vi "vaj timing control(new).vi"(8 "Error In":errorcluster, 10 "VAJ":cluster{"V":dbl, "A":dbl, "J":dbl}, 11 "D":dbl) -> (0 "Error Out":errorcluster, 3 "Array":cluster{"Numeric":dbl, "Numeric":dbl}[](array[cluster]))   [LabVIEW 2019]
uses:
  fd133df4-cac8-46f0-a5d4-c7e4d07d299a.vi
  2734163e-cfed-4914-b593-cf69aa2ffa15.vi
  <vilib>/Utility/error.llb/Error Cluster From Error Code.vi
  <vilib>/ErrorRing/Error Ring.xnode
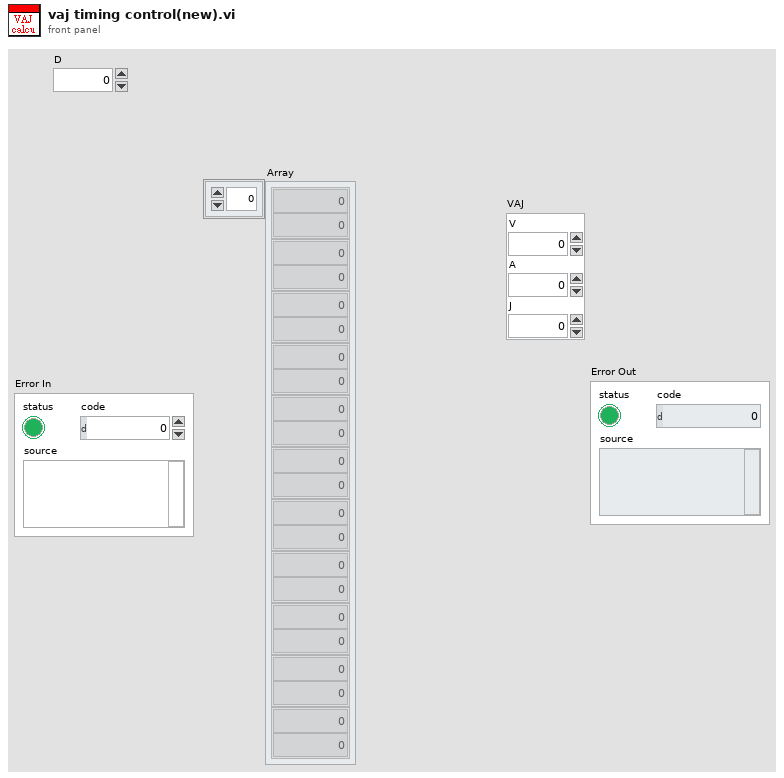
[diagram p1: front panel]
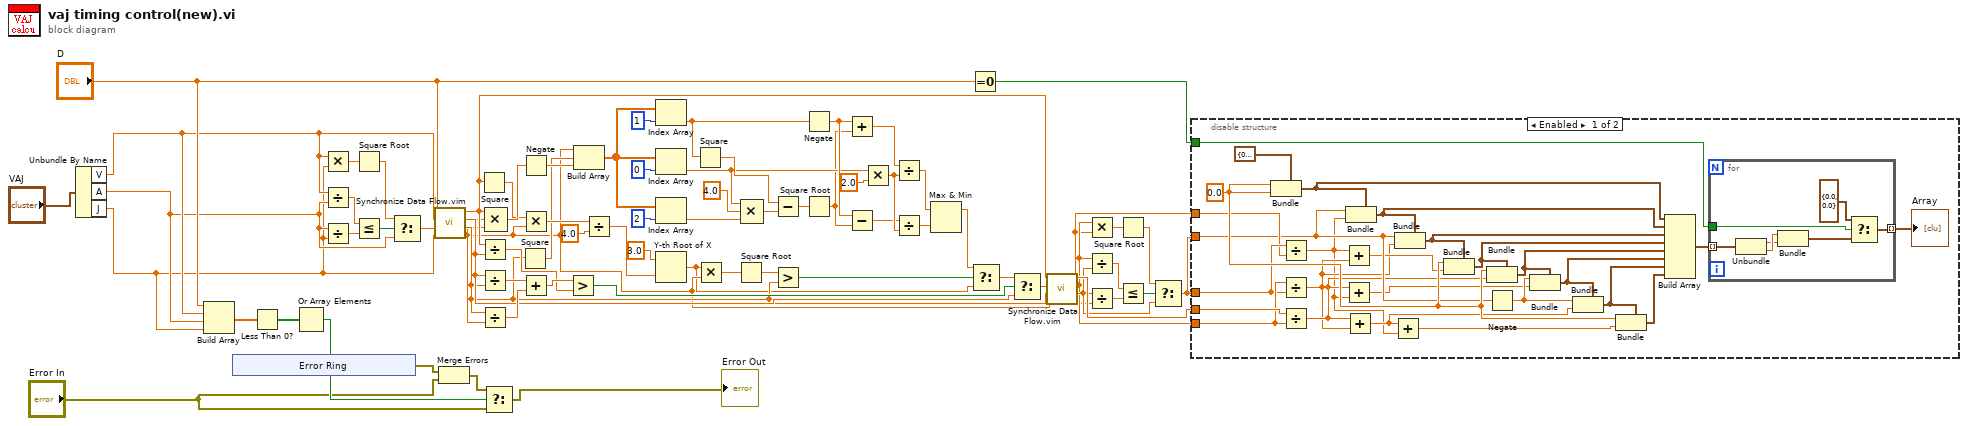
[diagram p0: block diagram]
diagram:
  n1 = Unbundle By Name("VAJ") -> ("V"=w10:dbl, "A"=w9:dbl, "J"=w8:dbl)
  n2 = Build Array("D", w10, w9, w8) -> (w7:dbl[])
  n3 = xnode "Error Ring"() -> ("error out"=w4:errorcluster)
  n4 = Less Than 0?(x=w7) -> (x < 0?=w6:bool[])
  n5 = Or Array Elements(Boolean array=w6) -> (logical OR=w5:bool)
  n6 = Multiply(x=w10, y=w8) -> (x*y=w69:dbl)
  n7 = Divide(x=w10, y=w9) -> (x/y=w72:dbl)
  n8 = Divide(x=w9, y=w8) -> (x/y=w71:dbl)
  n9 = Square Root(x=w69) -> (sqrt(x)=w68:dbl)
  n10 = Less Or Equal?(x=w72, y=w71) -> (x <= y?=w70:bool)
  n11 = Select(t=w68, s=w70, f=w9) -> (s? t:f=w67:dbl)
  n12 = call "Synchronize Data Flow.vim"("input 4"=w8, "input 3"=w67, "input 2"=w10, "input 1"="D") -> ("output 4"=w17:dbl, "output 3"=w18:dbl, "output 2"=w61:dbl, "output 1"=w29:dbl)
  n13 = Merge Errors(w4, "Error In") -> (w3:errorcluster)
  n14 = Square(x=w29) -> (x^2=w28:dbl)
  n15 = Divide(x=w29, y=w61) -> (x/y=w63:dbl)
  n16 = Divide(x=w61, y=w18) -> (x/y=w65:dbl)
  n17 = Divide(x=w18, y=w17) -> (x/y=w66:dbl)
  n18 = Select(t=w3, s=w5, f="Error In") -> (s? t:f=→"Error Out":errorcluster)
  n19 = Compound Arithmetic op=MULTIPLY(w29, w18, w17) -> (w60:dbl)
  n20 = Square(x=w18) -> (x^2=w19:dbl)
  n21 = Negate(x=w60) -> (-x=w59:dbl)
  n22 = Multiply(x=w28, y=w17) -> (x*y=w27:dbl)
  n23 = Add(x=w65, y=w66) -> (x+y=w64:dbl)
  n24 = Greater?(x=w64, y=w63) -> (0:w62:bool)
  n25 = Build Array(w17, w19, w59) -> (w55:dbl[])
  n26 = Divide(x=w27, y=4.0) -> (x/y=w25:dbl)
  n27 = Index Array(array=w55, index=1) -> (element=w49:dbl)
  n28 = Index Array(array=w55, index=0) -> (element=w46:dbl)
  n29 = Index Array(array=w55, index=2) -> (element=w45:dbl)
  n30 = Y-th Root of X(1:w25, 2:3.0 ("y")) -> (0:w16:dbl)
  n31 = Square(x=w49) -> (x^2=w48:dbl)
  n32 = Multiply(x=w16, y=w17) -> (x*y=w23:dbl)
  n33 = Square Root(x=w23) -> (sqrt(x)=w22:dbl)
  n34 = Compound Arithmetic op=MULTIPLY(w46, 4.0 ("value"), w45) -> (w47:dbl)
  n35 = Subtract(x=w48, y=w47) -> (x-y=w43:dbl)
  n36 = Greater?(x=w22, y=w18) -> (0:w21:bool)
  n37 = Negate(x=w49) -> (-x=w52:dbl)
  n38 = Square Root(x=w43) -> (sqrt(x)=w39:dbl)
  n39 = Add(x=w52, y=w39) -> (x+y=w51:dbl)
  n40 = Subtract(x=w52, y=w39) -> (x-y=w50:dbl)
  n41 = Multiply(x=w46, y=2.0) -> (x*y=w53:dbl)
  n42 = Divide(x=w51, y=w53) -> (x/y=w42:dbl)
  n43 = Divide(x=w50, y=w53) -> (x/y=w41:dbl)
  n44 = Max & Min(x=w42, y=w41) -> (max(x,y)=w20:dbl)  [unwired: 1 out]
  n45 = Equal To 0?(x="D") -> (x = 0?=w13:bool)
  n46 = Select(t=w20, s=w21, f=w16) -> (s? t:f=w15:dbl)
  n47 = Select(t=w15, s=w62, f=w61) -> (s? t:f=w14:dbl)
  n48 = call "Synchronize Data Flow.vim"("input 4"=w17, "input 3"=w18, "input 2"=w14, "input 1"=w29) -> ("output 4"=w31:dbl, "output 3"=w33:dbl, "output 2"=w32:dbl, "output 1"=w40:dbl)
  n49 = Multiply(x=w32, y=w31) -> (x*y=w35:dbl)
  n50 = Divide(x=w32, y=w33) -> (x/y=w38:dbl)
  n51 = Divide(x=w33, y=w31) -> (x/y=w37:dbl)
  n52 = Square Root(x=w35) -> (sqrt(x)=w34:dbl)
  n53 = Less Or Equal?(x=w38, y=w37) -> (x <= y?=w36:bool)
  n54 = Select(t=w34, s=w36, f=w33) -> (s? t:f=w30:dbl)
  n55 = disable-structure shown="Enabled" {
    disable-tunnel: w40 -> [w86 _]
    disable-tunnel: w32 -> [w85 _]
    disable-tunnel: w30 -> [w84 _]
    disable-tunnel: w31 -> [w83 _]
    disable-tunnel: w30 -> [w82 _]
    disable-tunnel: w13 -> [w73 _]
    frame Enabled {
      w95 = 0.0
      n56 = Bundle(cluster=cluster{dbl, dbl} {0.0, 0.0} ("output cluster"), w95, w95) -> (w93:cluster{dbl, dbl})
      n57 = Divide(x=w84, y=w83) -> (x/y=w74:dbl)
      n58 = Divide(x=w85, y=w84) -> (x/y=w77:dbl)
      n59 = Divide(x=w86, y=w85) -> (x/y=w78:dbl)
      n60 = Add(x=w74, y=w77) -> (x+y=w80:dbl)
      n61 = Add(x=w78, y=w74) -> (x+y=w79:dbl)
      n62 = Add(x=w78, y=w77) -> (x+y=w76:dbl)
      n63 = Bundle(cluster=w93, w82, w74) -> (w92:cluster{dbl, dbl})
      n64 = Add(x=w76, y=w74) -> (x+y=w75:dbl)
      n65 = Bundle(cluster=w92, w82, w77) -> (w91:cluster{dbl, dbl})
      n66 = Bundle(cluster=w91, w95, w80) -> (w90:cluster{dbl, dbl})
      n67 = Bundle(cluster=w90, w95, w78) -> (w89:cluster{dbl, dbl})
      n68 = Negate(x=w82) -> (-x=w81:dbl)
      n69 = Bundle(cluster=w89, w81, w79) -> (w88:cluster{dbl, dbl})
      n70 = Bundle(cluster=w88, w81, w76) -> (w87:cluster{dbl, dbl})
      n71 = Bundle(cluster=w87, w95, w75) -> (w98:cluster{dbl, dbl})
      n72 = Build Array(w93, w92, w91, w90, w89, w88, w87, w98) -> (w97:cluster{dbl, dbl}[])
      n73 = for {
        tunnel: w97 -> [w105] mode=indexing
        tunnel: [w102] -> w96 mode=indexing
        tunnel: w73 -> [w100]
        n74 = Unbundle(w105) -> (w103:dbl, w104:dbl)
        n75 = Bundle(w104, w103) -> (w101:cluster{dbl, dbl})  [unwired: 1 in]
        n76 = Select(t=cluster{dbl, dbl} {0.0, 0.0}, s=w100, f=w101) -> (s? t:f=w102:cluster{dbl, dbl})
      }
      "Array" <- w96
    }
    frame Disabled {
    }
  }
